vi "Viavi - prepSave.vi"(9 "Decimal Points":i32, 11 "Input Data":T1) -> (1 "Fail":bool, 2 "Data Output":string)   [LabVIEW 2017]
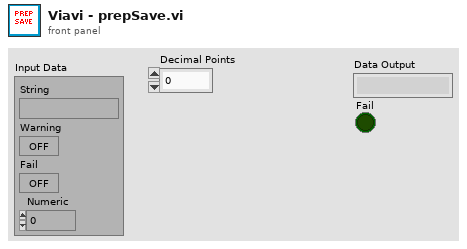
[diagram p1: front panel]
types:
  T1 = cluster{"String":string, "Warning":bool, "Fail":bool, "Numeric":dbl}
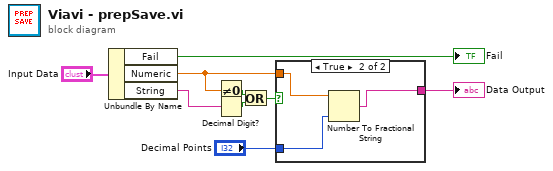
[diagram p0: block diagram]
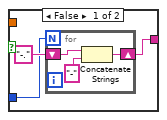
[diagram p2: hidden frame]
diagram:
  n1 = Unbundle By Name("Input Data") -> ("Fail"=→"Fail":bool, "Numeric"=w1:dbl, "String"=w5:string)
  n2 = Not Equal To 0?(x=w1) -> (x != 0?=w2:bool)
  n3 = Decimal Digit?(1:w5) -> (0:w3:bool)
  n4 = Or(x=w2, y=w3) -> (x .or. y?=w4:bool)
  n5 = case shown="True" w4 {
    tunnel: w1 -> [_ w18]
    tunnel: [w12 w17] -> w7
    tunnel: "Decimal Points" -> [w10 w16]
    frame False {
      n6 = for {
        N: w10 -> [_]
        shift-right: [w15] -> w12
        shift-left: "-." -> [w14]
        n7 = Concatenate Strings(w14, "-") -> (w15:string)
      }
    }
    frame True {
      n8 = Number To Fractional String(number=w18, precision (6)=w16) -> (F-format string=w17:string)  [unwired: 2 in]
    }
  }
  "Data Output" <- w7
